vi "PPS Close.vi"(8 "error in":errorcluster, 11 "IT-M6018C in":refnum<class "IT-M6018C.lvclass">) -> (0 "error out":errorcluster, 3 "IT-M6018C out":refnum<class "IT-M6018C.lvclass">)   [LabVIEW 2023, in "HardwareAbstractionLayer_LVOOP.lvlib" / "IT-M6018C.lvclass"]
uses:
  IT-M6018C.lvclass
  <instrlib>/IT6000C/IT6000C.lvlib
  PowerSupply.lvclass
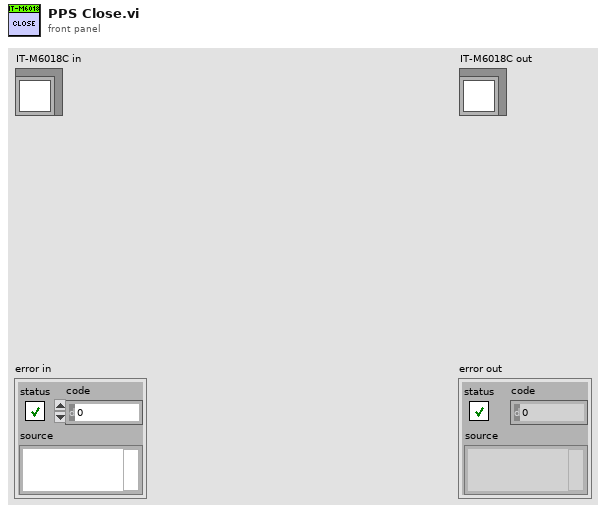
[diagram p1: front panel]
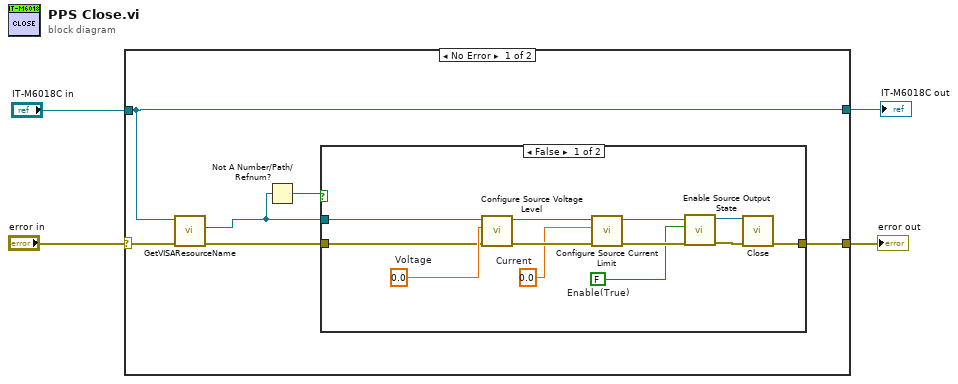
[diagram p0: block diagram]
diagram:
  n1 = case shown="No Error" "error in" {
    selector: "error in" -> [w9 w25]
    tunnel: [w10 w25] -> w3
    tunnel: "IT-M6018C in" -> [w7 w24]
    tunnel: [w7 w24] -> w1
    frame No Error {
      n2 = call "GetVISAResourceName.vi"("error in (no error)"=w9, "object in"=w7) -> ("error out"=w8:errorcluster, "VISA resource name"=w6:refnum<visa-resource-name>)  [unwired: 7 in, 1 out]
      n3 = Not A Number/Path/Refnum?(number/path/refnum=w6) -> (NaN/Path/Refnum?=w5:bool)
      n4 = case shown="False" w5 {
        tunnel: [w22 w23] -> w10
        tunnel: w8 -> [w12 w23]
        tunnel: w6 -> [w11 _]
        frame False {
          w13 = FALSE  # Enable(True)
          w14 = 0.0  # Current
          w15 = 0.0  # Voltage
          n5 = call <instrlib>:"Configure Source Voltage Level.vi"("error in (no error)"=w12, "Value(0)"=w15, "VISA resource name"=w11) -> ("error out"=w20:errorcluster, "VISA resource name out"=w21:refnum<visa-resource-name>)  [unwired: 7 in]
          n6 = call <instrlib>:"Configure Source Current Limit.vi"("error in (no error)"=w20, "Value(0)"=w14, "VISA resource name"=w21) -> ("error out"=w18:errorcluster, "VISA resource name out"=w19:refnum<visa-resource-name>)  [unwired: 7 in]
          n7 = call <instrlib>:"Enable Source Output State.vi"("error in (no error)"=w18, "Enable(True)"=w13, "VISA resource name"=w19) -> ("error out"=w17:errorcluster, "VISA resource name out"=w16:refnum<visa-resource-name>)  [unwired: 7 in]
          n8 = call <instrlib>:"Close.vi"("error in (no error)"=w17, "VISA resource name"=w16) -> ("error out"=w22:errorcluster)  [unwired: 9 in]
        }
        frame True {
        }
      }
    }
    frame Error {
    }
  }
  "error out" <- w3
  "IT-M6018C out" <- w1
